vi "EinGraph.vi"(1 "AIs":string[](array[string])) -> ()   [LabVIEW 2010]
uses:
  GVtdms.vi
  GVAbschalten.vi
panel:
  in  "Kombinationsfeld":string(combo)
  in  "JetztAbschalten":bool
  out "XY-Graph":cluster{dbl[], dbl[]}(graph)
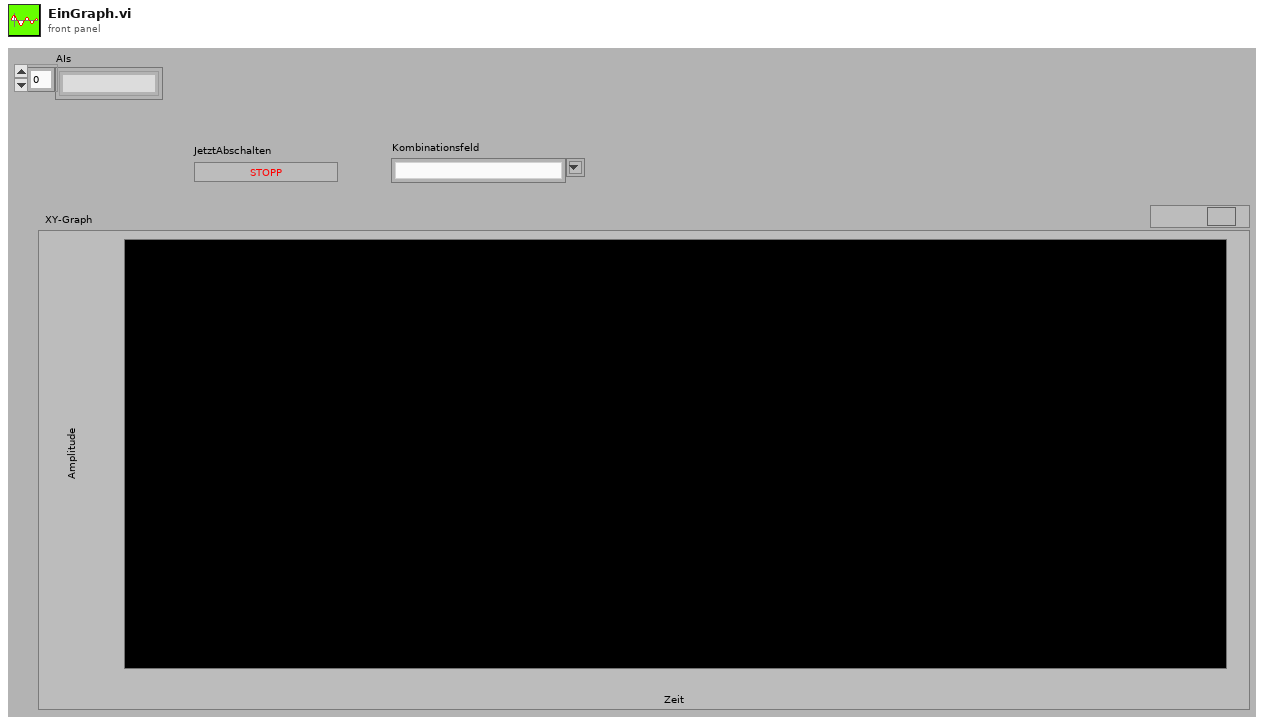
[diagram p1: front panel]
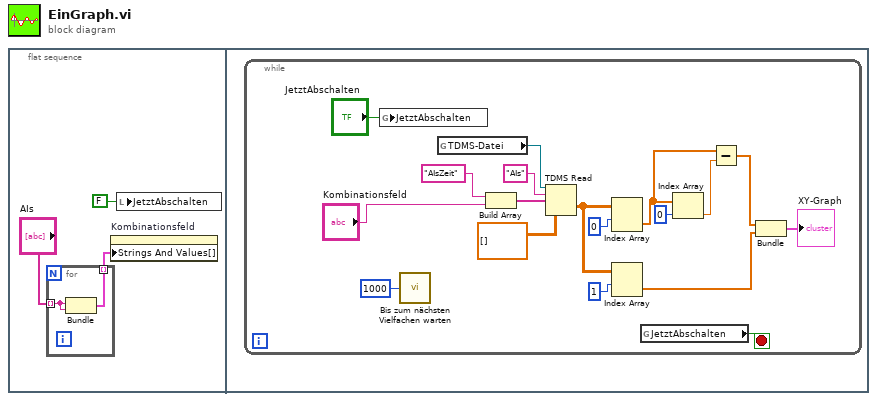
[diagram p0: block diagram]
diagram:
  n1 = flat-sequence {
    frame #0 {
      n2 = for {
        tunnel: "AIs" -> [w5] mode=indexing
        tunnel: [w4] -> w1 mode=indexing
        n3 = Bundle(w5, w5) -> (w4:cluster{string, string})  [unwired: 1 in]
      }
      n4 = property on="Kombinationsfeld" class="KombiFeld"("Strings And Values[]"=w1) -> ()  [unwired: 2 in, 2 out]
      n5 = local write "JetztAbschalten"(FALSE ("JetztAbschalten")) -> ()
    }
    frame #1 {
      n6 = while {
        stop <- w22 stop-if-true
        n7 = global write "GVAbschalten.vi" "JetztAbschalten"("JetztAbschalten") -> ()
        n8 = call "Bis zum nächsten Vielfachen warten"("Count(mSec)"=u32 1000) -> ()  [unwired: 1 out]
        n9 = global read "GVtdms.vi" "TDMS-Datei"() -> (w14:refnum<k34>)
        n10 = Build Array("AIsZeit", "Kombinationsfeld") -> (w19:string[])
        n11 = TDMS Read(0:w14, 5:"AIs" ("Gruppenname (Eingang)"), 7:w19, 12:dbl[][] []) -> (10:w17:dbl[][])  [unwired: 3 in, 5 out]
        n12 = Index Array(array=w17, index (row)=0 ("Deaktivierter Index (Spalte)")) -> (element=w9:dbl[])  [unwired: 1 in]
        n13 = Index Array(array=w17, index (row)=1 ("Deaktivierter Index (Spalte)")) -> (element=w16:dbl[])  [unwired: 1 in]
        n14 = global read "GVAbschalten.vi" "JetztAbschalten"() -> (w22:bool)
        n15 = Index Array(array=w9, index=0 ("Index")) -> (element=w7:dbl)
        n16 = Subtract(x=w9, y=w7) -> (x-y=w6:dbl[])
        n17 = Bundle(w6, w16) -> (→"XY-Graph":cluster{dbl[], dbl[]})  [unwired: 1 in]
      }
    }
  }
